vi "case.vi"(8 "Enum":enum16{"add", "sub", "mul", "div"}(ring), 10 "B":dbl, 11 "A":dbl) -> (3 "C":dbl)   [LabVIEW 2020]
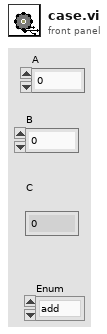
[diagram p1: front panel]
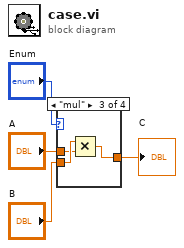
[diagram p0: block diagram]
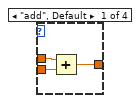
[diagram p2: hidden frame]
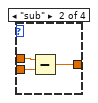
[diagram p3: hidden frame]
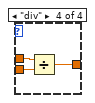
[diagram p4: hidden frame]
diagram:
  n1 = case shown="\"mul\"" "Enum" {
    tunnel: "A" -> [w7 w10 w12 w16]
    tunnel: "B" -> [w6 w9 w13 w15]
    tunnel: [w5 w8 w11 w14] -> w1
    frame "add", Default {
      n2 = Add(x=w7, y=w6) -> (x+y=w5:dbl)
    }
    frame "sub" {
      n3 = Subtract(x=w10, y=w9) -> (x-y=w8:dbl)
    }
    frame "mul" {
      n4 = Multiply(x=w13, y=w12) -> (x*y=w11:dbl)
    }
    frame "div" {
      n5 = Divide(x=w16, y=w15) -> (x/y=w14:dbl)
    }
  }
  "C" <- w1
